vi "2.analyse_fréquenciel.vi"() -> ()   [LabVIEW 2018]
uses:
  <vilib>/Analysis/4window.llb/windowTd.ctl
  <vilib>/measure/maspectr.llb/FFT Power Spectrum and PSD for 1 Chan.vi
  <vilib>/measure/maspectr.llb/FFT Spectrum (Mag-Phase) for 1 Chan.vi
  <vilib>/measure/NI_MABase.lvlib
  <vilib>/Analysis/NI_AALBase.lvlib
  <vilib>/measure/NI_MAPro.lvlib
  <vilib>/Analysis/NI_AALPro.lvlib
panel:
  out "Waveform Graph 2":waveform(dbl)(graph)
  in  "window":T1=1 items=["Rectangle"=0, "Hanning"=1, "Hamming"=2, "Blackman-Harris"=3, "Exact Blackman"=4, "Blackman"=5, "Flat Top"=6, "4 Term B-Harris "=7, "7 Term B-Harris"=8, "Low Sidelobe"=9, "Blackman Nuttall"=11, "Triangle"=30, "Bartlett-Hanning"=31, "Bohman"=32, "Parzen"=33, "Welch"=34, "Kaiser"=60, "Dolph-Chebyshev"=61, "Gaussian"=62]
  in  "Boolean":bool
  in  "nbr de signaux":dbl=2.0
  in  "stop":bool
  out "Waveform Graph":cluster{"f0":dbl, "df":dbl, "magnitude":dbl[]}(graph)
  in  "Amplitude":dbl=1.0
  in  "Paramétre de siganl 2":T2={"Fréquence Echantioll"=1000.0, "nombre des echantionnage"=1000.0}
  in  "Paramétre de siganl":T3={"Amplitude"=1.0, "frequence"=2.0, "signal type"=enum."Sine Wave"}
  # "Bruit"
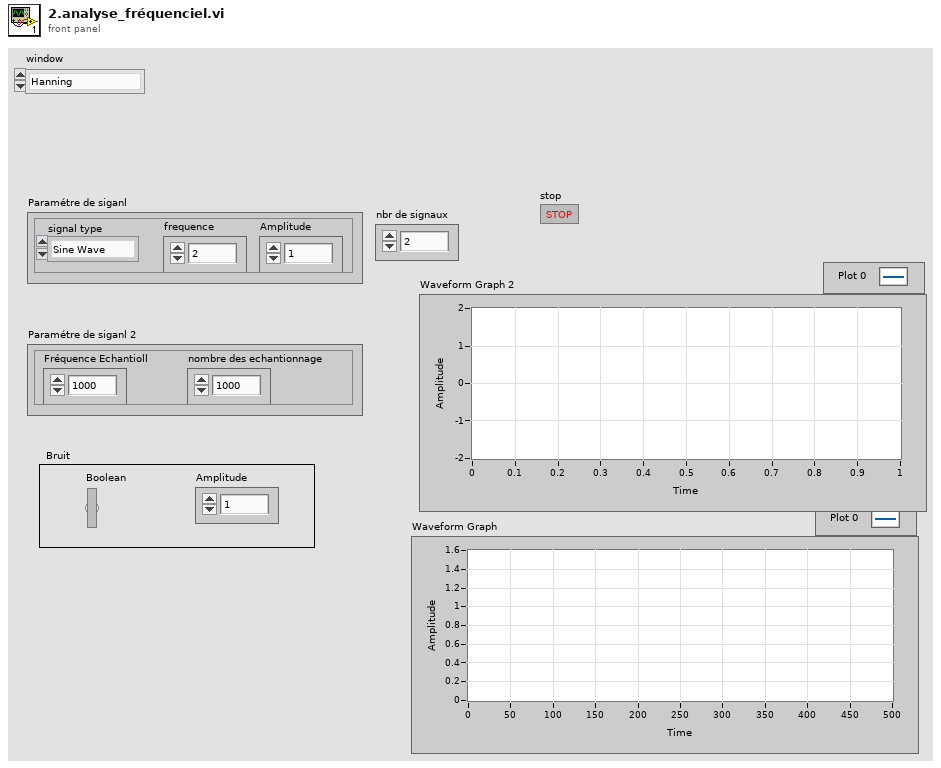
[diagram p1: front panel]
types:
  T1 = typedef "NI_AALPro.lvlib/windowTd.ctl" = u32
  T2 = cluster{"Fréquence Echantioll":dbl, "nombre des echantionnage":dbl}
  T3 = cluster{"Amplitude":dbl, "frequence":dbl, "signal type":enum16{"Sine Wave", "Triangle Wave", "Square Wave", "Sawtooth Wave"}}
  T4 = enum16{"Sine Wave", "Triangle Wave", "Square Wave", "Sawtooth Wave"}
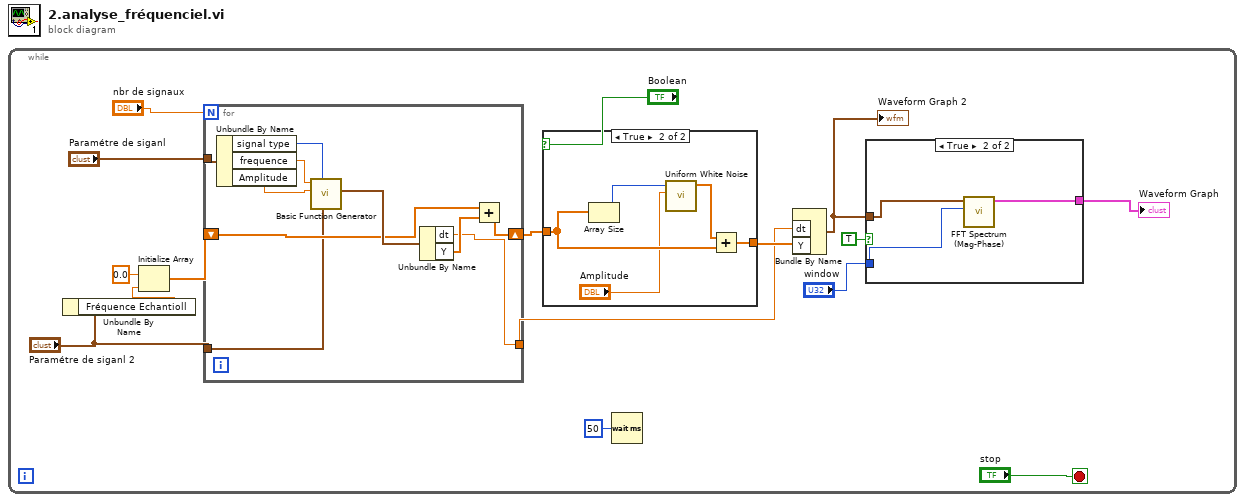
[diagram p0: block diagram]
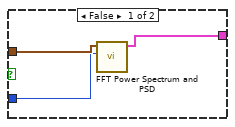
[diagram p2: hidden frame]
diagram:
  n1 = while {
    stop <- "stop" stop-if-true
    n2 = Unbundle By Name("Paramétre de siganl 2") -> ("Fréquence Echantioll"=w14:dbl)
    n3 = Initialize Array(0.0 ("element"), w14) -> (w16:dbl[])
    n4 = for {
      N: "nbr de signaux" -> [_]
      shift-right: [w36] -> w12
      shift-left: w16 -> [w35]
      tunnel: "Paramétre de siganl 2" -> [w34]
      tunnel: [w33] -> w10
      tunnel: "Paramétre de siganl" -> [w29]
      n5 = Unbundle By Name(w29) -> ("signal type"=w32:T4, "frequence"=w31:dbl, "Amplitude"=w30:dbl)
      n6 = call <vilib>:"Basic Function Generator.vi"("sampling info"=w34, "signal type"=w32, "amplitude"=w30, "frequency"=w31) -> ("signal out"=w38:waveform(dbl))  [unwired: 5 in, 2 out]
      n7 = Unbundle By Name(w38) -> ("dt"=w33:dbl, "Y"=w37:dbl[])
      n8 = Add(x=w35, y=w37) -> (x+y=w36:dbl[])
    }
    n9 = case shown="True" "Boolean" {
      tunnel: w12 -> [w23 w26]
      tunnel: [w23 w24] -> w11
      frame False {
      }
      frame True {
        n10 = Array Size(array=w26) -> (size(s)=w28:i32)
        n11 = call <vilib>:"Uniform White Noise.vi"("amplitude"="Amplitude", "samples"=w28) -> ("uniform white noise"=w27:dbl[])  [unwired: 8 in, 1 out]
        n12 = Add(x=w27, y=w26) -> (x+y=w24:dbl[])
      }
    }
    n13 = Wait (ms)(milliseconds to wait=u32 50) -> ()  [unwired: 1 out]
    n14 = Bundle By Name("dt"=w10, "Y"=w11) -> (w2:waveform(dbl))  [unwired: 1 in]
    "Waveform Graph 2" <- w2
    n15 = case shown="True" TRUE {
      tunnel: "window" -> [w17 w22]
      tunnel: w2 -> [w18 w21]
      tunnel: [w19 w20] -> w3
      frame False {
        n16 = call-poly <vilib>:"FFT Power Spectrum and PSD.vi"("window"=w17, "time signal"=w18) -> ("Power Spectrum / PSD"=w19:cluster{"f0":dbl, "df":dbl, "magnitude":dbl[]})  [unwired: 6 in, 3 out]
      }
      frame True {
        n17 = call-poly <vilib>:"FFT Spectrum (Mag-Phase).vi"("window"=w22, "time signal"=w21) -> ("magnitude"=w20:cluster{"f0":dbl, "df":dbl, "magnitude":dbl[]})  [unwired: 5 in, 4 out]
      }
    }
    "Waveform Graph" <- w3
  }
